vi "Get X from Re using calibration data (single point).vi"(1 "Calibration data":T1, 2 "Re":dbl) -> (0 "X":dbl format="%#_9g")   [LabVIEW 2022 SP3]
doc: "Get X = inv_f(Re) for a single point in Re using the calibration data.\nRoots of cubic spline equation.\nPN 15-OCT-24."
uses:
  Ctls/Calibration data.ctl
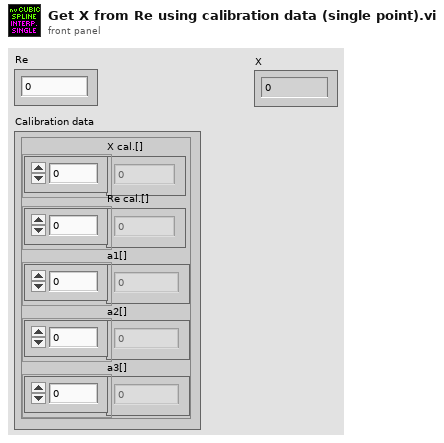
[diagram p1: front panel]
types:
  T1 = typedef "Calibration data.ctl" = cluster{"X cal.[]":dbl[], "Re cal.[]":dbl[], "a1[]":dbl[], "a2[]":dbl[], "a3[]":dbl[]}
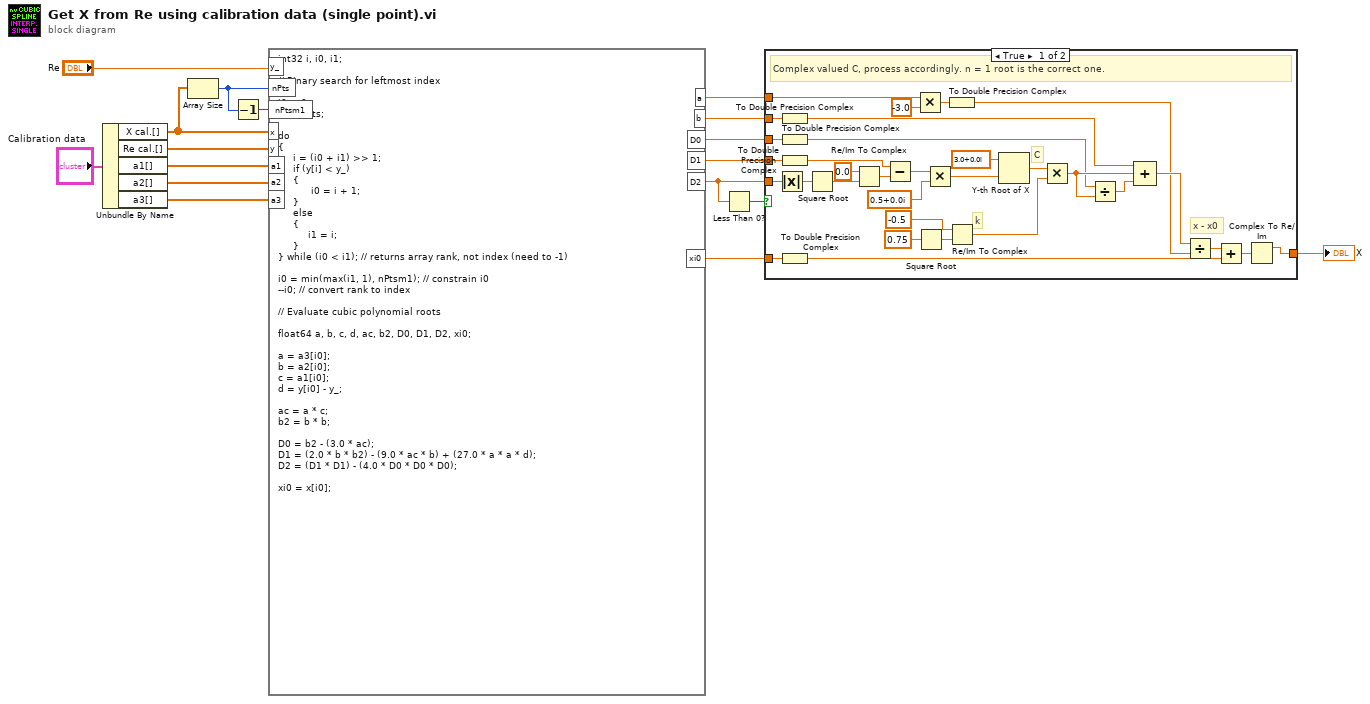
[diagram p0: block diagram]
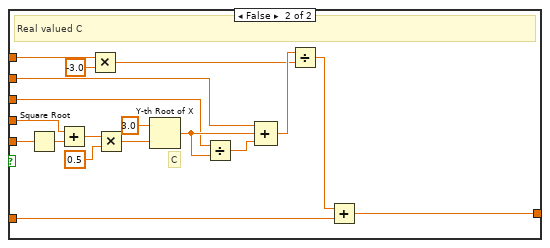
[diagram p2: hidden frame]
diagram:
  n1 = Unbundle By Name("Calibration data") -> ("X cal.[]"=w10:dbl[], "Re cal.[]"=w9:dbl[], "a1[]"=w13:dbl[], "a2[]"=w12:dbl[], "a3[]"=w11:dbl[])
  n2 = Array Size(array=w10) -> (size(s)=w16:i32)
  n3 = Decrement(x=w16) -> (x-1=w15:i32)
  n4 = formula code="int32 i, i0, i1;\n\n// Binary search for leftmost index\n\ni0 = 0;\ni1 = nPts;\n\ndo\n{\n     i = (i0 + i1) >> 1;\n     if (y[i] < y_)\n     {\n           i0 = i + 1;\n     }\n     else\n     {\n          i1 = i;\n     }\n} while (i0 < i1); // returns array rank, not index (need to -1)\n\ni0 = min(max(i1, 1), nPtsm1); // constrain i0\n--i0; // convert rank to index\n\n// Evaluate cubic polynomial roots\n\nfloat64 a, b, c, d, ac, b2, D0, D1, D2, xi0;\n\na = a3[i0];\nb = a2[i0];\nc = a1[i0];\nd = y[i0] - y_;\n\nac = a * c;\nb2 = b * b;\n\nD0 = b2 - (3.0 * ac);\nD1 = (2.0 * b * b2) - (9.0 * ac * b) + (27.0 * a * a * d);\nD2 = (D1 * D1) - (4.0 * D0 * D0 * D0);\n\nxi0 = x[i0];"("x"=w10, "nPts"=w16, "y_"="Re", "y"=w9, "nPtsm1"=w15, "a1"=w13, "a2"=w12, "a3"=w11) -> ("D2"=w3:dbl, "D1"=w8:dbl, "a"=w7:dbl, "b"=w6:dbl, "xi0"=w4:dbl, "D0"=w5:dbl)
  n5 = Less Than 0?(x=w3) -> (x < 0?=w2:bool)
  n6 = case shown="True" w2 {
    tunnel: w8 -> [w49 w52]
    tunnel: w7 -> [w23 w55]
    tunnel: w6 -> [w43 w54]
    tunnel: w5 -> [w41 w53]
    tunnel: w4 -> [w40 w56]
    tunnel: [w29 w57] -> w1
    tunnel: w3 -> [w28 w51]
    frame True {
      # "k"
      # "x - x0"
      # "C"
      # "Complex valued C, process accordingly. n = 1 root is the correct one."
      n7 = Absolute Value(x=w28) -> (abs(x)=w27:dbl)
      n8 = To Double Precision Complex(1:w43) -> (0:w35:cdb)
      n9 = To Double Precision Complex(1:w41) -> (0:w34:cdb)
      n10 = To Double Precision Complex(1:w49) -> (0:w48:cdb)
      n11 = To Double Precision Complex(1:w40) -> (0:w33:cdb)
      n12 = Square Root(x=w27) -> (sqrt(x)=w26:dbl)
      n13 = Re/Im To Complex(1:w26, 2:0.0 ("x")) -> (0:w25:cdb)
      n14 = Subtract(x=w48, y=w25) -> (x-y=w47:cdb)
      n15 = Multiply(x=w23, y=-3.0) -> (x*y=w18:dbl)
      n16 = Square Root(x=0.75 ("y")) -> (sqrt(x)=w20:dbl)
      n17 = Multiply(x=w47, y=cdb 0.5+0.0i) -> (x*y=w45:cdb)
      n18 = To Double Precision Complex(1:w18) -> (0:w22:cdb)
      n19 = Re/Im To Complex(1:w20, 2:-0.5 ("y")) -> (0:w19:cdb)
      n20 = Y-th Root of X(1:w45, 2:cdb 3.0+0.0i ("y")) -> (0:w30:cdb)
      n21 = Multiply(x=w30, y=w19) -> (x*y=w38:cdb)
      n22 = Divide(x=w34, y=w38) -> (x/y=w36:cdb)
      n23 = Compound Arithmetic op=ADD(w35, w38, w36) -> (w37:cdb)
      n24 = Divide(x=w37, y=w22) -> (x/y=w32:cdb)
      n25 = Add(x=w32, y=w33) -> (x+y=w31:cdb)
      n26 = Complex To Re/Im(x + iy=w31) -> (x=w29:dbl)  [unwired: 1 out]
    }
    frame False {
      # "C"
      # "Real valued C"
      n27 = Square Root(x=w51) -> (sqrt(x)=w67:dbl)
      n28 = Add(x=w52, y=w67) -> (x+y=w66:dbl)
      n29 = Multiply(x=w55, y=-3.0) -> (x*y=w50:dbl)
      n30 = Multiply(x=w66, y=0.5) -> (x*y=w64:dbl)
      n31 = Y-th Root of X(1:w64, 2:3.0 ("y")) -> (0:w58:dbl)
      n32 = Divide(x=w53, y=w58) -> (x/y=w61:dbl)
      n33 = Compound Arithmetic op=ADD(w54, w58, w61) -> (w60:dbl)
      n34 = Divide(x=w60, y=w50) -> (x/y=w59:dbl)
      n35 = Add(x=w59, y=w56) -> (x+y=w57:dbl)
    }
  }
  "X" <- w1
